vi "Lookup Channel DBL.vi"(8 "error in (no error)":errorcluster, 10 "Name":string, 11 "VolatusAPI in":refnum<class "VolatusAPI.lvclass">) -> (0 "error out":errorcluster, 2 "Channel DBL":refnum<class "Channel DBL.lvclass">, 3 "VolatusAPI out":refnum<class "VolatusAPI.lvclass">)   [LabVIEW 2020, in "Volatus.lvlib" / "VolatusAPI.lvclass"]
uses:
  VolatusAPI.lvclass
  lv-vecto/Vecto/Channel DBL/Channel DBL.lvclass
  VolatusAPI.lvclass/VolatusAPI.ctl
  lv-vecto/Vecto/ChannelService/ChannelService.lvclass
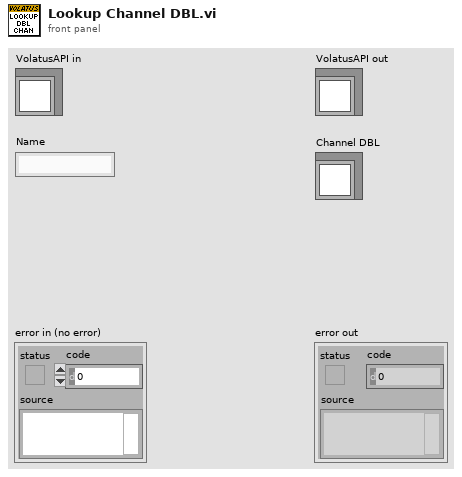
[diagram p1: front panel]
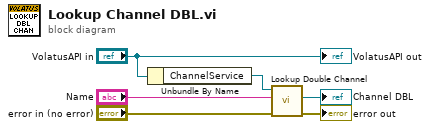
[diagram p0: block diagram]
diagram:
  n1 = Unbundle By Name("VolatusAPI in") -> ("ChannelService"=w5:refnum<class "ChannelService.lvclass">)
  n2 = call "Lookup Double Channel.vi"("error in (no error)"="error in (no error)", "Channel Name"="Name", "ChannelService in"=w5) -> ("error out"=→"error out":errorcluster, "Channel"=→"Channel DBL":refnum<class "Channel DBL.lvclass">)  [unwired: 6 in, 1 out]
  "VolatusAPI out" <- "VolatusAPI in"
